vi "MODBUS_IonGauge.vi"(8 "error in":errorcluster, 10 "unit ID":u8, 11 "Modbus instance in":refnum<class "Modbus Master.lvclass">) -> (0 "error out":errorcluster, 1 "Pirani":sgl, 2 "Ion Gauge Pressure":sgl, 3 "Modbus instance out":refnum<class "Modbus Master.lvclass">)   [LabVIEW 2016]
uses:
  <vilib>/NI/Modbus Library/API/Master/Modbus Master.lvclass
  C:/Program Files (x86)/National Instruments/LabVIEW 2016/vi.lib/NI/Modbus Library/API/Modbus API.lvclass
  <vilib>/NI/Modbus Library/API/Modbus API.lvclass/Modbus API.ctl
  <vilib>/NI/Modbus Library/Transmission Data Unit/Transmission Data Unit.lvclass/Transmission Data Unit.ctl
  <vilib>/NI/Modbus Library/Transmission Data Unit/Write Unit ID.vi
  <vilib>/NI/Modbus Library/API/Read Transmission Data Unit.vi
  <vilib>/NI/Modbus Library/API/Write Transmission Data Unit.vi
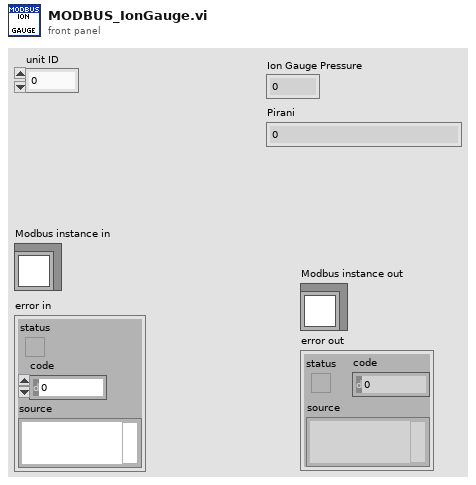
[diagram p1: front panel]
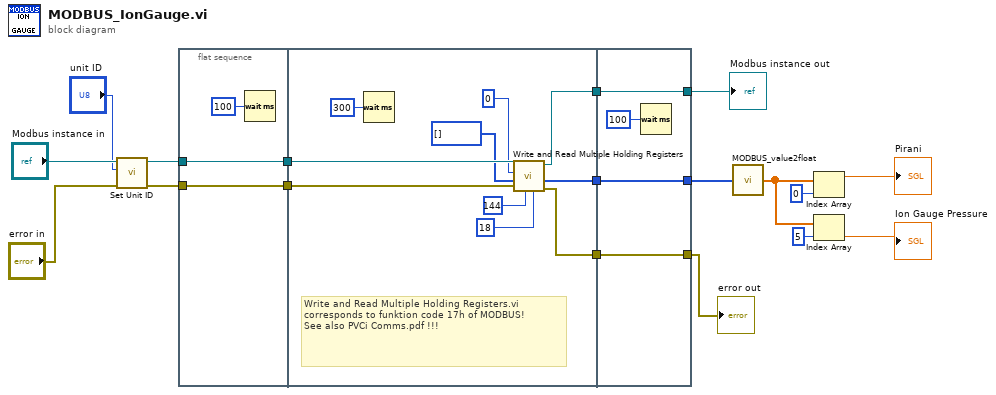
[diagram p0: block diagram]
diagram:
  n1 = call <vilib>:"Set Unit ID.vi"("error in"="error in", "unit ID"="unit ID", "Modbus master in"="Modbus instance in") -> ("error out"=w16:errorcluster, "Modbus master out"=w17:refnum<class "Modbus Master.lvclass">)  [unwired: 7 in]
  n2 = flat-sequence {
    tunnel: w16 -> [w20]
    tunnel: w17 -> [w21]
    tunnel: [w21] -> w6
    tunnel: [w20] -> w5
    tunnel: w6 -> [w30]
    tunnel: w5 -> [w29]
    tunnel: [w31] -> w3
    tunnel: [w28] -> w2
    tunnel: [w27] -> w1
    tunnel: [w33] -> w4
    tunnel: [w34] -> w12
    tunnel: [w35] -> w18
    tunnel: w3 -> [w35]
    tunnel: w2 -> [w34]
    tunnel: w1 -> [w33]
    frame #0 {
      n3 = Wait (ms)(milliseconds to wait=u32 100) -> ()  [unwired: 1 out]
    }
    frame #1 {
      # "Write and Read Multiple Holding Registers.vi corresponds to funktion code 17h of MODBUS!\nSee also PVCi Comms.pdf !!!"
      n4 = Wait (ms)(milliseconds to wait=u32 300) -> ()  [unwired: 1 out]
      n5 = call-dynamic "Write and Read Multiple Holding Registers.vi"("read count"=u16 18, "read starting address"=u16 144, "error in"=w29, "write values"=u16[] [], "write starting address"=u16 0, "Modbus instance in"=w30) -> ("error out"=w27:errorcluster, "read values"=w31:u16[], "Modbus instance out"=w28:refnum<class "Modbus Master.lvclass">)  [unwired: 3 in]
    }
    frame #2 {
      n6 = Wait (ms)(milliseconds to wait=u32 100) -> ()  [unwired: 1 out]
    }
  }
  n7 = call "MODBUS_value2float.vi"("MODBUS parameter"=w18) -> ("float"=w10:sgl[])
  n8 = Index Array(array=w10, index=0) -> (element=→"Pirani":sgl)
  n9 = Index Array(array=w10, index=5) -> (element=→"Ion Gauge Pressure":sgl)
  "Modbus instance out" <- w12
  "error out" <- w4
